vi "Turn.vi"(7 "PID gains":T5={"proportional gain (Kc)"=1.0, "integral time (Ti, min)"=0.0, "derivative time (Td, min)"=0.0}, 8 "Right MotorControlDevRef in":T1={"DeviceStatus"={"status"=FALSE, "code"=0, "source"=""}, "Type"=enum."PWM", "PWM"={"PWM Channel"=enum."Invalid", "DeadBand"={"Name"="", "maxPositivePwm"=0, "minPositivePwm"=0, "centerPwm"=0, "maxNegativePwm"=0, "minNegativePwm"=0, "angularRange"=0}}, "CAN"={"Device Number"=0, "SetOutput VI Ref"=variant(refnum<vi> refnum), "GetOutput VI Ref"=variant(refnum<vi> refnum), "Enable VI Ref"=variant(refnum<vi> refnum), "Disable VI Ref"=variant(refnum<vi> refnum), "Data"=variant}, "Invert"=FALSE}, 9 "Left MotorControlDevRef in":T1={"DeviceStatus"={"status"=FALSE, "code"=0, "source"=""}, "Type"=enum."PWM", "PWM"={"PWM Channel"=enum."Invalid", "DeadBand"={"Name"="", "maxPositivePwm"=0, "minPositivePwm"=0, "centerPwm"=0, "maxNegativePwm"=0, "minNegativePwm"=0, "angularRange"=0}}, "CAN"={"Device Number"=0, "SetOutput VI Ref"=variant(refnum<vi> refnum), "GetOutput VI Ref"=variant(refnum<vi> refnum), "Enable VI Ref"=variant(refnum<vi> refnum), "Disable VI Ref"=variant(refnum<vi> refnum), "Data"=variant}, "Invert"=FALSE}, 11 "Gyro target":dbl) -> (0 "Right MotorControlDevRef out":T1={"DeviceStatus"={"status"=FALSE, "code"=0, "source"=""}, "Type"=enum."PWM", "PWM"={"PWM Channel"=enum."Invalid", "DeadBand"={"Name"="", "maxPositivePwm"=0, "minPositivePwm"=0, "centerPwm"=0, "maxNegativePwm"=0, "minNegativePwm"=0, "angularRange"=0}}, "CAN"={"Device Number"=0, "SetOutput VI Ref"=variant(refnum<vi> refnum), "GetOutput VI Ref"=variant(refnum<vi> refnum), "Enable VI Ref"=variant(refnum<vi> refnum), "Disable VI Ref"=variant(refnum<vi> refnum), "Data"=variant}, "Invert"=FALSE}, 1 "Left MotorControlDevRef out":T1={"DeviceStatus"={"status"=FALSE, "code"=0, "source"=""}, "Type"=enum."PWM", "PWM"={"PWM Channel"=enum."Invalid", "DeadBand"={"Name"="", "maxPositivePwm"=0, "minPositivePwm"=0, "centerPwm"=0, "maxNegativePwm"=0, "minNegativePwm"=0, "angularRange"=0}}, "CAN"={"Device Number"=0, "SetOutput VI Ref"=variant(refnum<vi> refnum), "GetOutput VI Ref"=variant(refnum<vi> refnum), "Enable VI Ref"=variant(refnum<vi> refnum), "Disable VI Ref"=variant(refnum<vi> refnum), "Data"=variant}, "Invert"=FALSE}, 3 "Turn time out":u32, 6 "Yaw out":dbl)   [LabVIEW 2016]
uses:
  <vilib>/Rock Robotics/WPI/MotorControl/WPI_MotorControlDeviceRef.ctl
  <vilib>/Rock Robotics/WPI/MotorControl/WPI_MotorControlType.ctl
  <vilib>/Rock Robotics/SystemInterfaces/DIO/FPGA_DIOPWMChannel.ctl
  <vilib>/Rock Robotics/WPI/PWM/WPI_PWMDeadband.ctl
  <vilib>/Rock Robotics/WPI/ThirdParty/CanMotor/TalonSRX/WPI_CANTalonSRX_APIControlMode.ctl
  <vilib>/addons/control/pid/pid.llb/PID (DBL).vi
  <vilib>/addons/control/pid/NI_PID_pid.lvlib
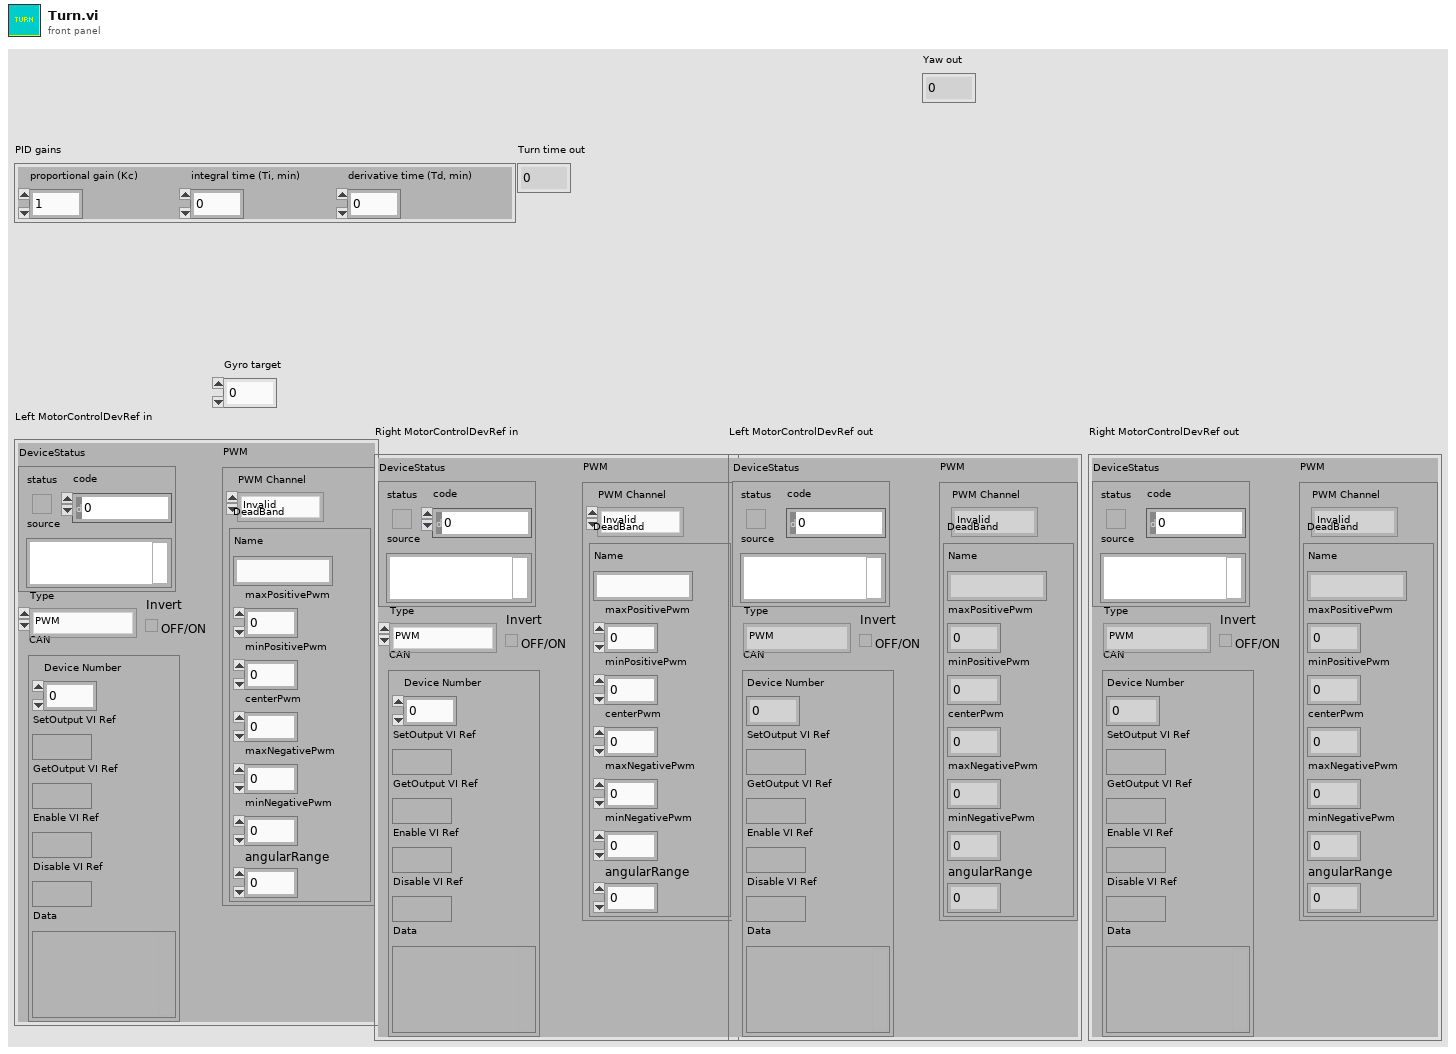
[diagram p1: front panel]
types:
  T1 = typedef "WPI_MotorControlDeviceRef.ctl" = cluster{"DeviceStatus":errorcluster, "Type":T2, "PWM":cluster{"PWM Channel":T3, "DeadBand":T4}, "CAN":cluster{"Device Number":u8, "SetOutput VI Ref":variant, "GetOutput VI Ref":variant, "Enable VI Ref":variant, "Disable VI Ref":variant, "Data":variant}, "Invert":bool}
  T2 = typedef "WPI_MotorControlType.ctl" = enum16{"PWM", "CAN"}
  T3 = typedef "FPGA_DIOPWMChannel.ctl" = enum8{"PWM 0", "PWM 1", "PWM 2", "PWM 3", "PWM 4", "PWM 5", "PWM 6", "PWM 7", "PWM 8", "PWM 9", "PWM MXP 0", "PWM MXP 1", "PWM MXP 2", "PWM MXP 3", "PWM MXP 4", "PWM MXP 5", "PWM MXP 6", "PWM MXP 7", "PWM MXP 8", "PWM MXP 9", "Invalid"}
  T4 = typedef "WPI_PWMDeadband.ctl" = cluster{"Name":string, "maxPositivePwm":i32, "minPositivePwm":i32, "centerPwm":i32, "maxNegativePwm":i32, "minNegativePwm":i32, "angularRange":u16}
  T5 = cluster{"proportional gain (Kc)":dbl, "integral time (Ti, min)":dbl, "derivative time (Td, min)":dbl}
  T6 = typedef "WPI_CANTalonSRX_APIControlMode.ctl" = enum8{"Percent VBus", "Speed", "Position", "Slave", "Unchanged / Invalid", "Voltage Compensation", "Current", "Motion Profile", "Motion Magic"}
  T7 = cluster{"Yaw":dbl, "Roll":dbl, "Pitch":dbl, "Heading":dbl, "Fused Heading":dbl}
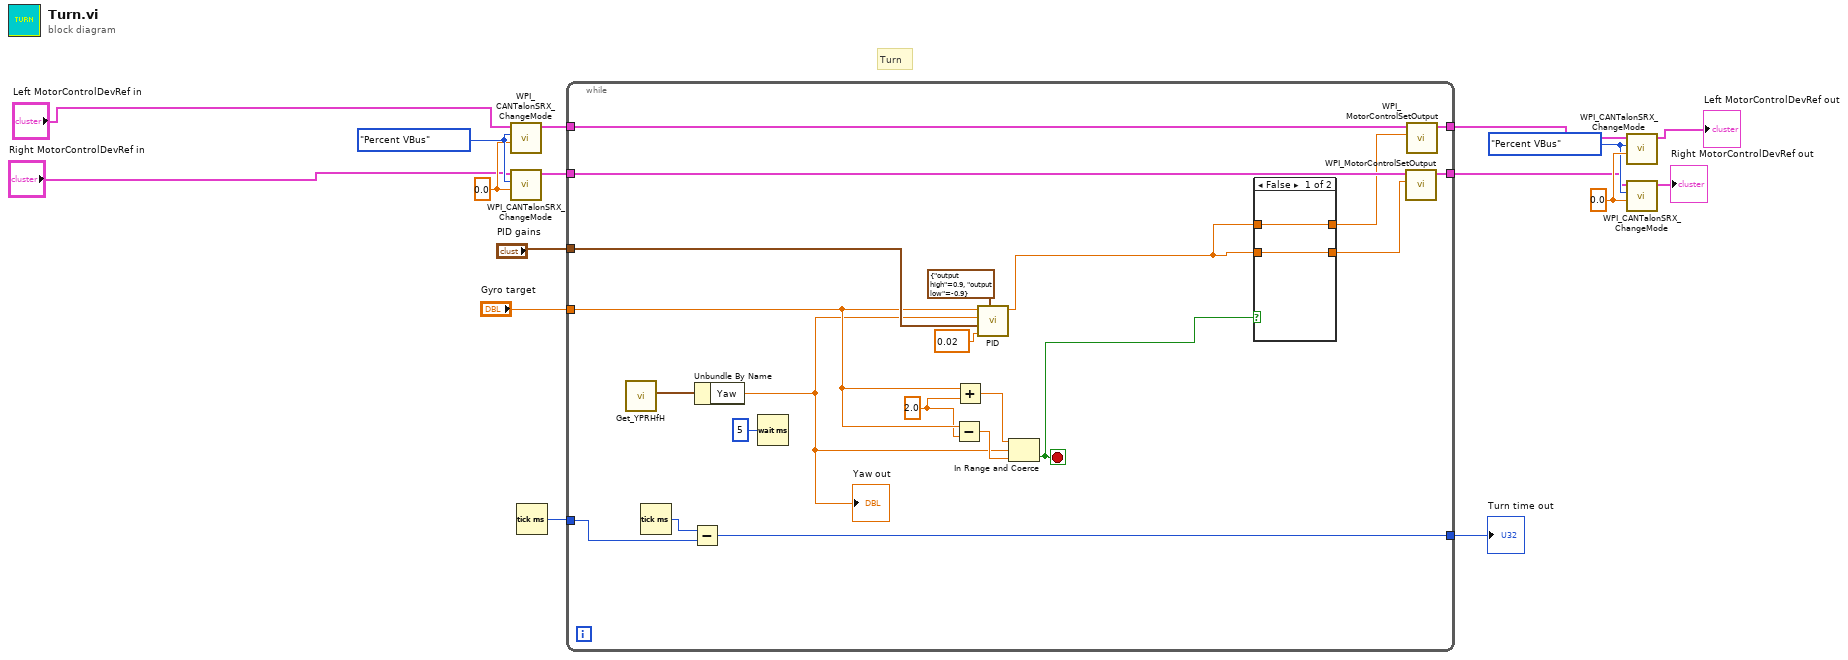
[diagram p0: block diagram]
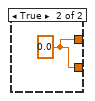
[diagram p2: hidden frame]
diagram:
  w10 = 0.0
  w9 = WPI_CANTalonSRX_APIControlMode."Percent VBus" ("Control Mode")
  w13 = 0.0
  w14 = WPI_CANTalonSRX_APIControlMode."Percent VBus" ("Control Mode")
  # "Turn"
  n1 = call <vilib>:"WPI_CANTalonSRX_ChangeMode.vi"("Output"=w13, "Control Mode"=w14, "CAN Talon SRX Ref"="Left MotorControlDevRef in") -> ("CAN Talon SRX Ref"=w12:T1)  [unwired: 7 in, 1 out]
  n2 = call <vilib>:"WPI_CANTalonSRX_ChangeMode.vi"("Output"=w13, "Control Mode"=w14, "CAN Talon SRX Ref"="Right MotorControlDevRef in") -> ("CAN Talon SRX Ref"=w11:T1)  [unwired: 7 in, 1 out]
  n3 = Tick Count (ms)() -> (millisecond timer value=w6:u32)
  n4 = while {
    tunnel: "PID gains" -> [w35]
    tunnel: "Gyro target" -> [w34]
    tunnel: w12 -> [w29]
    tunnel: w11 -> [w28]
    tunnel: [w27] -> w8
    tunnel: [w26] -> w7
    tunnel: w6 -> [w25]
    tunnel: [w19] -> w1
    stop <- w21 stop-if-true
    w33 = 2.0
    n5 = call <vilib>:"Get_YPRHfH.vi"() -> ("YRPHfH"=w18:T7)  [unwired: 11 in]
    n6 = Tick Count (ms)() -> (millisecond timer value=w24:u32)
    n7 = Subtract(x=w24, y=w25) -> (x-y=w19:u32)
    n8 = Unbundle By Name(w18) -> ("Yaw"=w17:dbl)
    "Yaw out" <- w17
    n9 = Wait (ms)(milliseconds to wait=u32 5) -> ()  [unwired: 1 out]
    n10 = Subtract(x=w34, y=w33) -> (x-y=w31:dbl)
    n11 = Add(x=w34, y=w33) -> (x+y=w32:dbl)
    n12 = call-poly <vilib>:"PID.vi"("output range"=cluster{"output high":dbl, "output low":dbl} {"output high"=0.9, "output low"=-0.9}, "dt (s)"=0.02, "PID gains"=w35, "process variable"=w17, "setpoint"=w34) -> ("output"=w20:dbl)  [unwired: 5 in, 1 out]
    n13 = In Range and Coerce(upper limit=w32, x=w17, lower limit=w31) -> (In Range?=w21:bool)  [unwired: 1 out]
    n14 = case shown="False" w21 {
      tunnel: w20 -> [w39 _]
      tunnel: w20 -> [w38 _]
      tunnel: [w39 w40] -> w22
      tunnel: [w38 w40] -> w23
      frame False {
      }
      frame True {
        w40 = 0.0
      }
    }
    n15 = call <vilib>:"WPI_MotorControlSetOutput.vi"("Output"=w23, "MotorControlDevRef"=w28) -> ("MotorControlDevRef"=w26:T1)  [unwired: 7 in, 2 out]
    n16 = call <vilib>:"WPI_MotorControlSetOutput.vi"("Output"=w22, "MotorControlDevRef"=w29) -> ("MotorControlDevRef"=w27:T1)  [unwired: 7 in, 2 out]
  }
  "Turn time out" <- w1
  n17 = call <vilib>:"WPI_CANTalonSRX_ChangeMode.vi"("Output"=w10, "Control Mode"=w9, "CAN Talon SRX Ref"=w8) -> ("CAN Talon SRX Ref"=→"Left MotorControlDevRef out":T1)  [unwired: 7 in, 1 out]
  n18 = call <vilib>:"WPI_CANTalonSRX_ChangeMode.vi"("Output"=w10, "Control Mode"=w9, "CAN Talon SRX Ref"=w7) -> ("CAN Talon SRX Ref"=→"Right MotorControlDevRef out":T1)  [unwired: 7 in, 1 out]
